vi "SR Number Comparison.vi"(8 "SR Cluster 2 in":T1 {"Creation Date" format="%<%x>T"; "Last Updated" format="%<%x>T"}, 9 "SR Cluster 1 in":T1 {"Creation Date" format="%<%x>T"; "Last Updated" format="%<%x>T"}, 10 "flip? in":bool, 11 "equal? in":bool=TRUE) -> (0 "SR Cluster 2 out":T1 {"Creation Date" format="%<%x>T"; "Last Updated" format="%<%x>T"}, 1 "SR Cluster 1 out":T1 {"Creation Date" format="%<%x>T"; "Last Updated" format="%<%x>T"}, 2 "flip? out":bool, 3 "equal? out":bool)   [LabVIEW 2018]
uses:
  Type Defs/SR Cluster.ctl
  Type Defs/SR Status.ctl
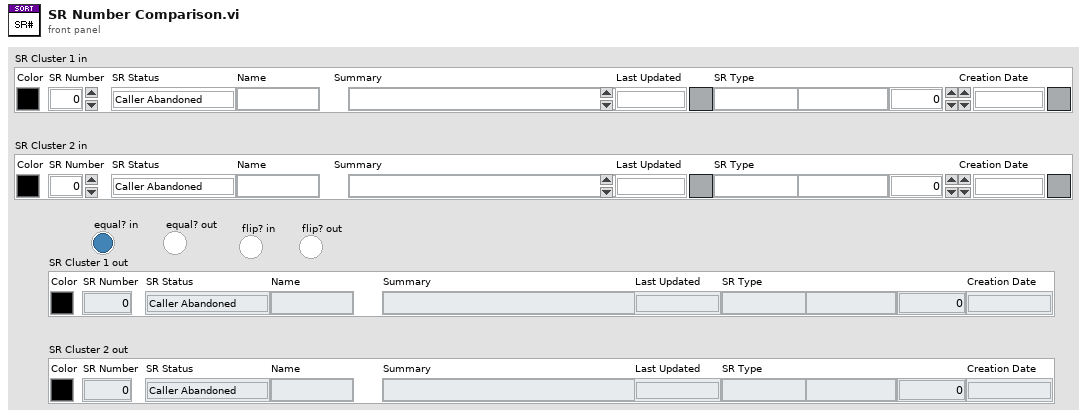
[diagram p1: front panel]
types:
  T1 = typedef "SR Cluster.ctl" = cluster{"Color":u32, "SR Number":i32, "SR Status":T2, "Name":string, "Summary":string, "Last Updated":timestamp, "SR Type":string, "Service Level":string, "Days Open":dbl, "Creation Date":timestamp}
  T2 = typedef "SR Status.ctl" = enum16{"Caller Abandoned", "Created in Error", "Expired", "Forum Resolved AE", "Forum Resolved Customer", "IN WORK", "IN WORK Collab with AES", "IN WORK Collab with PSE", "IN WORK Collab with SE", "IN WORK Customer Added Note", "IN WORK Escalation", "IN WORK Wait on Customer", "Open", "Potentially Resolved", "Presumed Resolved", "RMA Approved for Return", "Resolved", "Passed Off"}
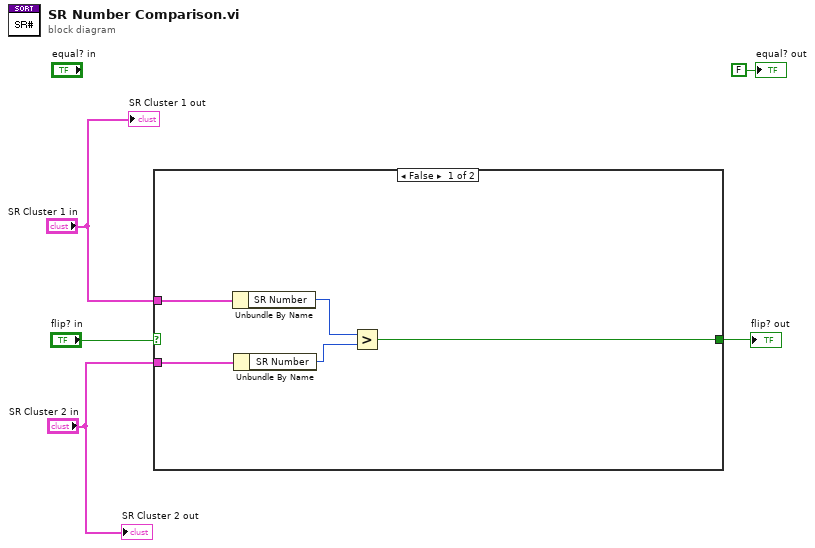
[diagram p0: block diagram]
diagram:
  n1 = case shown="False" "flip? in" {
    selector: "flip? in" -> [_ w11]
    tunnel: [w8 w11] -> w4
    tunnel: "SR Cluster 2 in" -> [w7 _]
    tunnel: "SR Cluster 1 in" -> [w6 _]
    frame False {
      n2 = Unbundle By Name(w6) -> ("SR Number"=w9:i32)
      n3 = Unbundle By Name(w7) -> ("SR Number"=w10:i32)
      n4 = Greater?(x=w9, y=w10) -> (0:w8:bool)
    }
    frame True {
    }
  }
  "flip? out" <- w4
  "equal? out" <- FALSE ("equal? out")
  "SR Cluster 2 out" <- "SR Cluster 2 in"
  "SR Cluster 1 out" <- "SR Cluster 1 in"
